vi "Number_of_trues.vi"(11 "Boolean Array":bool[](array[boolean])) -> (3 "Number of True Values":i32)   [LabVIEW 2016]
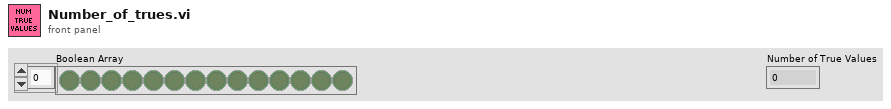
[diagram p1: front panel]
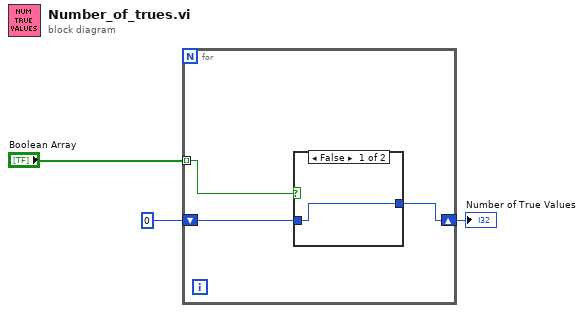
[diagram p0: block diagram]
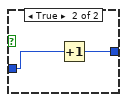
[diagram p2: hidden frame]
diagram:
  n1 = for {
    tunnel: "Boolean Array" -> [w6] mode=indexing
    shift-right: [w4] -> w1
    shift-left: 0 -> [w5]
    n2 = case shown="False" w6 {
      tunnel: w5 -> [w7 w9]
      tunnel: [w7 w8] -> w4
      frame False {
      }
      frame True {
        n3 = Increment(x=w9) -> (x+1=w8:i32)
      }
    }
  }
  "Number of True Values" <- w1
